vi "命令转换.vi"(11 "启动命令":T1) -> (3 "控制命令":T2, 5 "布尔":bool)   [LabVIEW 2016, in "ZK定时设置.xctl"]
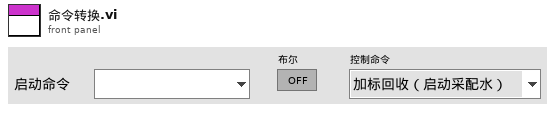
[diagram p1: front panel]
types:
  T1 = typedef "ZK定时设置.xctl/启动命令选择.ctl" = enum16{"", "加标回收（启动采配水）", "加标回收（不启动采配水）", "水样测试（启动采配水）", "水样测试（不启动采配水）"}
  T2 = typedef "ZK定时设置.xctl/国标控制命令.ctl" = enum16{"加标回收（启动采配水）", "加标回收（不启动采配水）", "水样测试（启动采配水）", "水样测试（不启动采配水）"}
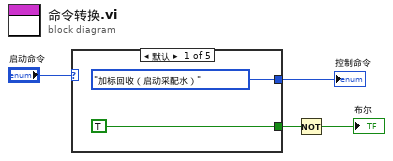
[diagram p0: block diagram]
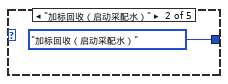
[diagram p2: hidden frame]
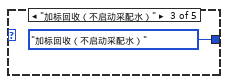
[diagram p3: hidden frame]
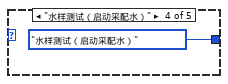
[diagram p4: hidden frame]
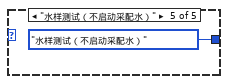
[diagram p5: hidden frame]
diagram:
  n1 = case shown="默认" "启动命令" {
    tunnel: [国标控制命令."加标回收（启动采配水）" ("控制命令") 国标控制命令."加标回收（启动采配水）" ("控制命令") 国标控制命令."加标回收（不启动采配水）" ("控制命令") 国标控制命令."水样测试（启动采配水）" ("控制命令") 国标控制命令."水样测试（不启动采配水）" ("控制命令")] -> w2
    tunnel: [TRUE _ _ _ _] -> w3
    frame Default {
    }
    frame "加标回收（启动采配水）" {
    }
    frame "加标回收（不启动采配水）" {
    }
    frame "水样测试（启动采配水）" {
    }
    frame "水样测试（不启动采配水）" {
    }
  }
  "控制命令" <- w2
  n2 = Not(x=w3) -> (.not. x?=→"布尔":bool)
